vi "Setup PID.vi"() -> ()   [LabVIEW 2019]
uses:
  Controls/Global - Data UDP.vi
  Controls/UDP - Command.ctl
  Controls/Communication - Write Data.ctl
panel:
  in  "IP Address":string
  in  "Set":bool
  in  "Get":bool
  in  "Tab Control":enum32{"System", "Test", "ADC", "Sensor", "PID"}(tab)
  in  "System":string[][](table)=[["Out_Type"], ["Inverse"], ["Monitor"], ["ACC_Time"], ["Pulse_rev"], ["Stroke"], ["Auto Off"], ["Gear_Ratio"], ["Pitch"], ["Max Speed"], ["Jog Speed"], ["Disp Coff"], ["Max Load"]]
  in  "Test":string[][](table)=[["Traget #1"], ["Target #2"], ["Speed #1"], ["Speed #2"], [""], [""], [""], [""], [""], [""], [""], [""]]
  in  "ADC":string[][](table)=[["ActiveCH #0"], ["ActiveCH #1"], ["ActiveCH #2"], ["ActiveCH #3"], ["ActiveCH #4"], ["ActiveCH #5"], ["ActiveCH #6"], ["ActiveCH #7"], ["FilterType"], ["PostFilter #0"], ["PostFilter #1"], ["PostFilter #2"], ["PostFilter #3"], ["PostFilter #4"], ["PostFilter #5"], ["PostFilter #6"], ["PostFilter #7"], ["Gain #0"], ["Gain #1"], ["Gain #2"], ["Gain #3"], ["Gain #4"], ["Gain #5"], ["Gain #6"], ["Gain #7"], ["FS"], ["IntOC"], ["IntFC"], ["SysOC"], ["Cofficient #0"], ["Cofficient #1"], ["Cofficient #2"], ["Cofficient #3"], ["Cofficient #4"], ["Cofficient #5"], ["Cofficient #6"], ["Cofficient #7"], ["K1"], ["K2"], ["Max"]]
  in  "Sensor":string[][](table)=[["#1", ""], ["Name", ""], ["SUnit", ""], ["DecPoint", ""], ["Log", ""], ["H_Alarm", ""], ["L_Alarm", ""], ["H_Limit", ""], ["L_Limit", ""], ["Filter", ""], ["Gain", ""], ["Cal Type", " "], ["", ""], ["#2", ""], ["Name", ""], ["SUnit", ""], ["DecPoint", ""], ["Log", ""], ["H_Alarm", ""], ["L_Alarm", ""], ["H_Limit", ""], ["L_Limit", ""], ["Filter", ""], ["Gain", ""], ["Cal Type", ""], ["", ""], ["#3", ""], ["Name", ""], ["SUnit", ""], ["DecPoint", ""], ["Log", ""], ["H_Alarm", ""], ["L_Alarm", ""], ["H_Limit", ""], ["L_Limit", ""], ["Filter", ""], ["Gain", ""], ["Cal Type", ""], ["", ""], ["#4", ""], ["Name", ""], ["SUnit", ""], ["DecPoint", ""], ["Log", ""], ["H_Alarm", ""], ["L_Alarm", ""], ["H_Limit", ""], ["L_Limit", ""], ["Filter", ""], ["Gain", ""], ["Cal Type", ""]]
  in  "PID":string[][](table)=[["SP"], ["PV"], ["KP"], ["KI"], ["KD"], ["FF"], ["Err_Band"], ["Max"], ["Min"], ["Ts"], ["Out"], ["Mode"]]
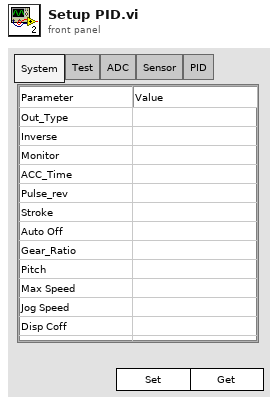
[diagram p1: front panel]
types:
  T1 = typedef "Communication - Write Data.ctl" = cluster{"Test":cluster{"Target Load":sgl, "Target Disp":sgl, "Rate":sgl, "Speed":sgl}, "Sensor":cluster{"Name":string[], "Unit":string[], "Decimal Point":u8[], "Ch Log":u8[], "H Alarm":u8[], "L Alarm":u8[], "H Limit":sgl[], "L Limit":sgl[], "Filter":u8[], "Gain":u8[], "Calib Type":u32[]}, "PID":cluster{"SP":sgl, "PV":sgl, "kP":sgl, "kI":sgl, "kD":sgl, "FF":sgl, "Err Band":sgl, "Max":i32, "Min":i32, "Ts":u32, "Out":i32, "Mode":u8}, "ADC":cluster{"Active Ch":u8[], "Filter Type":u8, "Post Filter":u8[], "Gain":u8[], "FS":u16, "IntOC":u8, "IntFC":u8, "SysOC":u8, "Cofficient":dbl[], "K":dbl[], "Max":i32}, "System":cluster{"Out Type":u8, "Inverse":u8, "Monitor":u8, "Reserve":u8, "ACC Time":u32, "Pulse Rev":u32, "Stroke":u32, "Auto Off":u32, "Gear Ratio":sgl, "Pitch":sgl, "Max Speed":u32, "Jog Speed":u32, "Disp Coff":sgl, "Max Load":u32}, "Index":enum16{"Ch1", "Ch2", "Ch3", "Ch4", "Ch5", "Ch6", "Ch7", "Ch8", "Ch9", "Ch10", "Ch11", "Ch12", "Ch13", "Ch14", "Ch15", "Ch16"}, "Datalog":enum16{"Ch1-Ch16", "Ch17-Ch32", "Ch32-Ch48", "Ch49-Ch64", "Empty"}}
  T2 = enum16{"Init", "Idle", "Get System", "Get Test", "Get ADC", "Get Sensor", "Get PID", "Set System", "Set Test", "Set ADC", "Set Sensor", "Set PID", "Exit"}
  T3 = typedef "UDP - Command.ctl" = enum16{"Stop", "Jog Up", "Jog Down", "Ramp Up", "Ramp Down", "PID Target", "PID Ramp", "Disp Run", "Read Ch Data", "Zero Channel", "Zero Disp", "Read Sensor", "Write Sensor", "Read ADC", "Write ADC", "Read PID", "Write PID", "Read Test", "Write Test", "Read System", "Write System", "Read Datalog", "Read Datalog Sensor"}
  T4 = cluster{"Out Type":u8, "Inverse":u8, "Monitor":u8, "Reserve":u8, "ACC Time":u32, "Pulse Rev":u32, "Stroke":u32, "Auto Off":u32, "Gear Ratio":sgl, "Pitch":sgl, "Max Speed":u32, "Jog Speed":u32, "Disp Coff":sgl, "Max Load":u32}
  T5 = cluster{"Out Type":string, "Inverse":string, "Monitor":string, "Reserve":string, "ACC Time":string, "Pulse Rev":string, "Stroke":string, "Auto Off":string, "Gear Ratio":string, "Pitch":string, "Max Speed":string, "Jog Speed":string, "Disp Coff":string, "Max Load":string}
  T6 = cluster{"Target Load":sgl, "Target Disp":sgl, "Rate":sgl, "Speed":sgl}
  T7 = cluster{"Target Load":string, "Target Disp":string, "Rate":string, "Speed":string}
  T8 = cluster{"Active Ch":u8[], "Filter Type":u8, "Post Filter":u8[], "Gain":u8[], "FS":u16, "IntOC":u8, "IntFC":u8, "SysOC":u8, "Cofficient":dbl[], "K":dbl[], "Max":i32}
  T9 = cluster{"Name":string[], "Unit":string[], "Decimal Point":u8[], "Ch Log":u8[], "H Alarm":u8[], "L Alarm":u8[], "H Limit":sgl[], "L Limit":sgl[], "Filter":u8[], "Gain":u8[], "Calib Type":u32[]}
  T10 = cluster{"SP":sgl, "PV":sgl, "kP":sgl, "kI":sgl, "kD":sgl, "FF":sgl, "Err Band":sgl, "Max":i32, "Min":i32, "Ts":u32, "Out":i32, "Mode":u8}
  T11 = cluster{"SP":string, "PV":string, "kP":string, "kI":string, "kD":string, "FF":string, "Err Band":string, "Max":string, "Min":string, "Ts":string, "Out":string, "Mode":string}
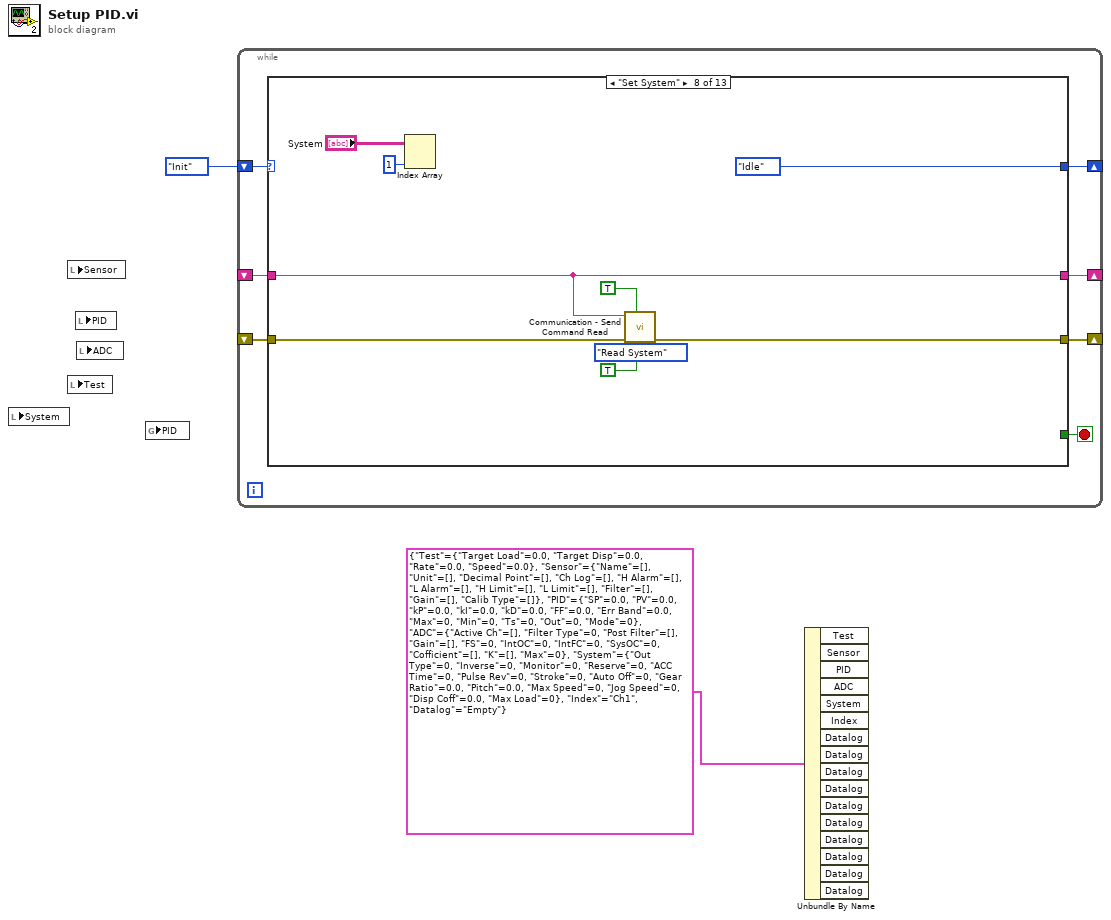
[diagram p0: block diagram]
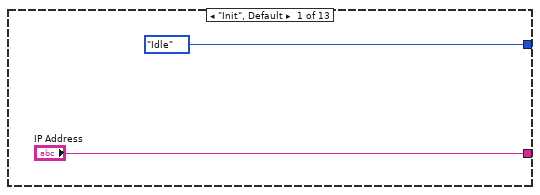
[diagram p2: hidden frame]
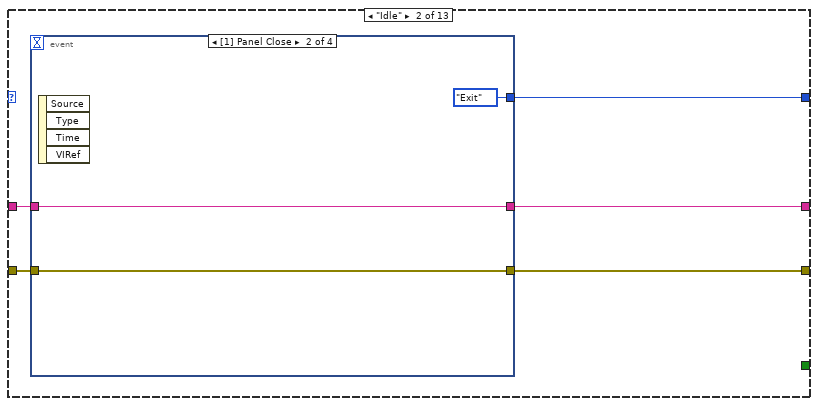
[diagram p3: hidden frame]
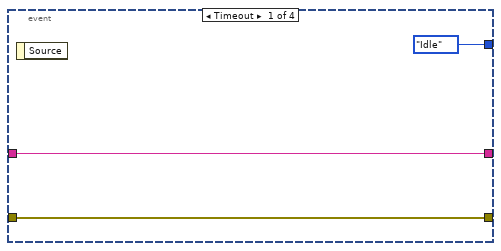
[diagram p4: hidden frame]
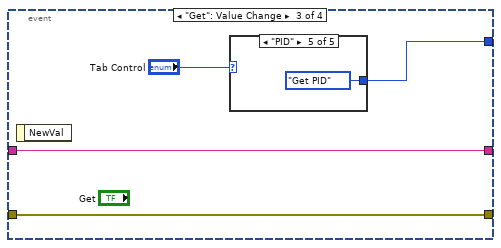
[diagram p5: hidden frame]
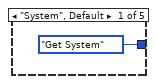
[diagram p6: hidden frame]
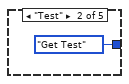
[diagram p7: hidden frame]
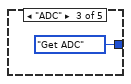
[diagram p8: hidden frame]
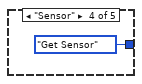
[diagram p9: hidden frame]
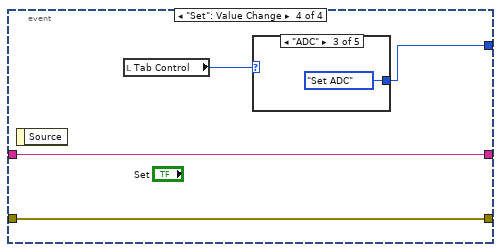
[diagram p10: hidden frame]
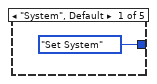
[diagram p11: hidden frame]
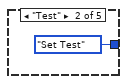
[diagram p12: hidden frame]
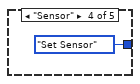
[diagram p13: hidden frame]
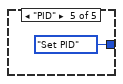
[diagram p14: hidden frame]
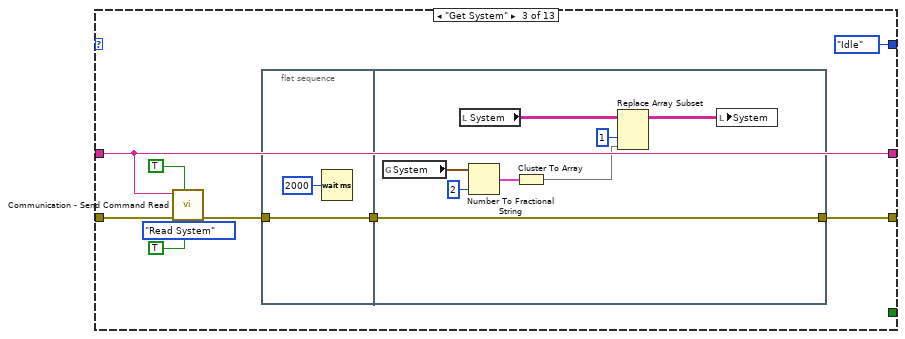
[diagram p15: hidden frame]
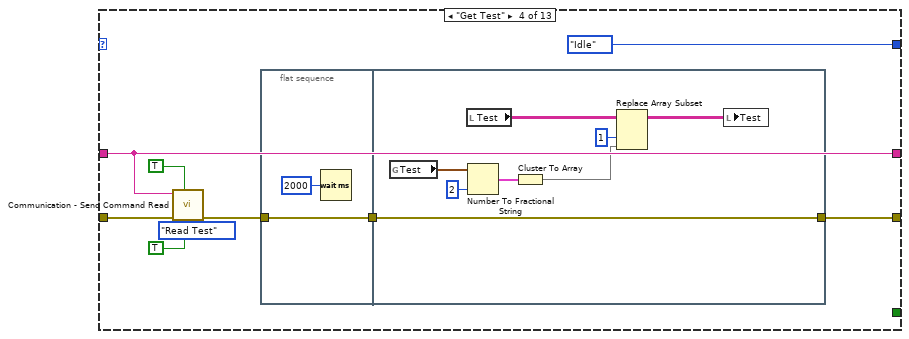
[diagram p16: hidden frame]
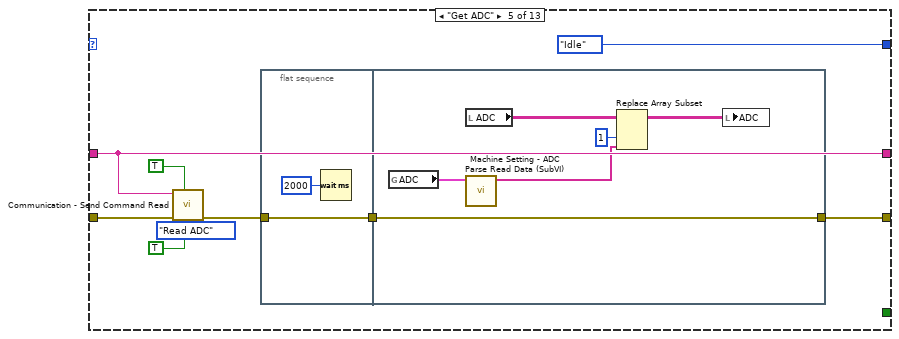
[diagram p17: hidden frame]
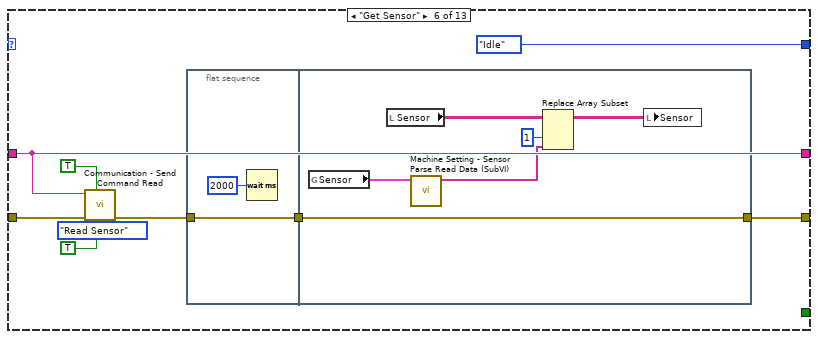
[diagram p18: hidden frame]
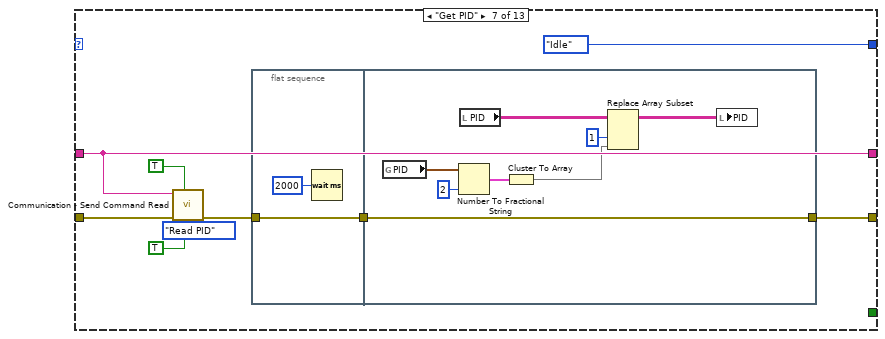
[diagram p19: hidden frame]
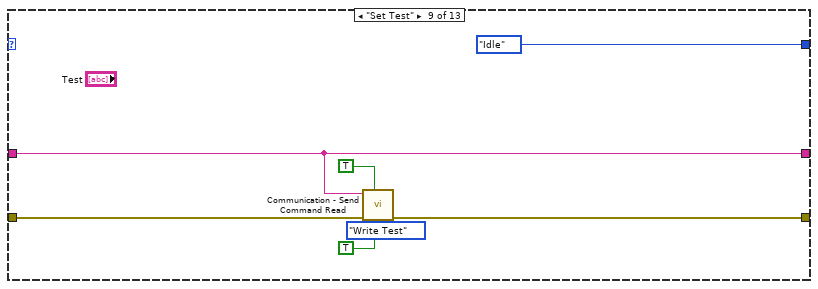
[diagram p20: hidden frame]
diagram:
  n1 = local read "System"() -> ()  [unwired: 1 in]
  n2 = local read "Sensor"() -> ()  [unwired: 1 in]
  n3 = local read "Test"() -> ()  [unwired: 1 in]
  n4 = local read "PID"() -> ()  [unwired: 1 in]
  n5 = local read "ADC"() -> ()  [unwired: 1 in]
  n6 = global read "Global - Data UDP.vi" "PID"() -> ()  [unwired: 1 in]
  n7 = while {
    shift-right: [w8] -> _
    shift-left: T2."Init" -> [w9]
    shift-right: [w6] -> _
    shift-left: _ -> [w5]
    shift-right: [w4] -> _
    shift-left: _ -> [w3]
    stop <- w7 stop-if-true
    n8 = case shown="\"Set System\"" w9 {
      tunnel: [T2."Idle" w16 T2."Idle" T2."Idle" T2."Idle" T2."Idle" T2."Idle" T2."Idle" T2."Idle" T2."Idle" T2."Idle" T2."Idle" T2."Exit"] -> w8
      tunnel: [_ _ _ _ _ _ _ _ _ _ _ _ TRUE] -> w7
      tunnel: ["IP Address" w14 w46 w63 w82 w99 w116 w134 w141 w148 w155 w162 "" ("IP Address")] -> w6
      tunnel: w5 -> [_ w15 w46 w63 w82 w99 w116 w134 w141 w148 w155 w162 _]
      tunnel: [_ w13 w43 w60 w79 w96 w113 w135 w142 w149 w156 w163 _] -> w4
      tunnel: w3 -> [_ w12 w47 w64 w83 w100 w117 w136 w143 w150 w157 w164 _]
      frame "Init", Default {
      }
      frame "Idle" {
        n9 = event shown="[1] Panel Close" {
          selector: _ -> [_ _ _ _]
          dyn-events: _ -> [_ _ _ _]
          timeout: _ -> [_ _ _ _]
          tunnel: [T2."Idle" T2."Exit" w25 w34] -> w16
          tunnel: w15 -> [w18 w22 w24 w33]
          tunnel: [w18 w22 w24 w33] -> w14
          tunnel: [w17 w20 w23 w32] -> w13
          tunnel: w12 -> [w17 w20 w23 w32]
          event Timeout {
            n10 = event-data() -> ()  [unwired: 1 in, 1 out]
          }
          event Panel Close {
            n11 = event-data() -> ()  [unwired: 1 in, 4 out]
          }
          event "Get": Value Change {
            n12 = event-data() -> ()  [unwired: 1 in, 1 out]
            n13 = case shown="\"PID\"" "Tab Control" {
              tunnel: [T2."Get System" T2."Get Test" T2."Get ADC" T2."Get Sensor" T2."Get PID"] -> w25
              frame "System", Default {
              }
              frame "Test" {
              }
              frame "ADC" {
              }
              frame "Sensor" {
              }
              frame "PID" {
              }
            }
          }
          event "Set": Value Change {
            n14 = event-data() -> ()  [unwired: 1 in, 1 out]
            n15 = local read "Tab Control"() -> (w35:enum32{"System", "Test", "ADC", "Sensor", "PID"})
            n16 = case shown="\"ADC\"" w35 {
              tunnel: [T2."Set System" T2."Set Test" T2."Set ADC" T2."Set Sensor" T2."Set PID"] -> w34
              frame "System", Default {
              }
              frame "Test" {
              }
              frame "ADC" {
              }
              frame "Sensor" {
              }
              frame "PID" {
              }
            }
          }
        }
      }
      frame "Get System" {
        n17 = call "Communication - Send Command Read.vi"("Fron?"=TRUE, "Bypass?"=TRUE, "error in (no error)"=w47, "Action"=UDP_-_Command."Read System", "Device IP Address"=w46) -> ("error out"=w41:errorcluster)  [unwired: 6 in]
        n18 = flat-sequence {
          tunnel: [w50] -> w42
          tunnel: w41 -> [w50]
          tunnel: [w52] -> w43
          tunnel: w42 -> [w52]
          frame #0 {
            n19 = Wait (ms)(milliseconds to wait=u32 2000) -> ()  [unwired: 1 out]
          }
          frame #1 {
            n20 = global read "Global - Data UDP.vi" "System"() -> (w56:T4)
            n21 = local read "System"() -> (w59:string[][])
            n22 = Number To Fractional String(number=w56, precision (6)=i16 2) -> (F-format string=w54:T5)  [unwired: 2 in]
            n23 = Cluster To Array(cluster=w54) -> (array=w53:string[])
            n24 = Replace Array Subset(array=w59, new element=w53, index (col)=1 ("disabled index (col)")) -> (w58:string[][])  [unwired: 1 in]
            n25 = local write "System"(w58) -> ()
          }
        }
      }
      frame "Get Test" {
        n26 = call "Communication - Send Command Read.vi"("Fron?"=TRUE, "Bypass?"=TRUE, "error in (no error)"=w64, "Action"=UDP_-_Command."Read Test", "Device IP Address"=w63) -> ("error out"=w61:errorcluster)  [unwired: 6 in]
        n27 = flat-sequence {
          tunnel: [w69] -> w62
          tunnel: w61 -> [w69]
          tunnel: [w71] -> w60
          tunnel: w62 -> [w71]
          frame #0 {
            n28 = Wait (ms)(milliseconds to wait=u32 2000) -> ()  [unwired: 1 out]
          }
          frame #1 {
            n29 = global read "Global - Data UDP.vi" "Test"() -> (w75:T6)
            n30 = local read "Test"() -> (w78:string[][])
            n31 = Number To Fractional String(number=w75, precision (6)=i16 2) -> (F-format string=w73:T7)  [unwired: 2 in]
            n32 = Cluster To Array(cluster=w73) -> (array=w72:string[])
            n33 = Replace Array Subset(array=w78, new element=w72, index (col)=1 ("disabled index (col)")) -> (w77:string[][])  [unwired: 1 in]
            n34 = local write "Test"(w77) -> ()
          }
        }
      }
      frame "Get ADC" {
        n35 = call "Communication - Send Command Read.vi"("Fron?"=TRUE, "Bypass?"=TRUE, "error in (no error)"=w83, "Action"=UDP_-_Command."Read ADC", "Device IP Address"=w82) -> ("error out"=w80:errorcluster)  [unwired: 6 in]
        n36 = flat-sequence {
          tunnel: [w88] -> w81
          tunnel: w80 -> [w88]
          tunnel: [w92] -> w79
          tunnel: w81 -> [w92]
          frame #0 {
            n37 = Wait (ms)(milliseconds to wait=u32 2000) -> ()  [unwired: 1 out]
          }
          frame #1 {
            n38 = global read "Global - Data UDP.vi" "ADC"() -> (w91:T8)
            n39 = local read "ADC"() -> (w95:string[][])
            n40 = call "Machine Setting - ADC Parse Read Data (SubVI).vi"("ADC"=w91) -> ("Array"=w90:string[])  [unwired: 10 in]
            n41 = Replace Array Subset(array=w95, new element=w90, index (col)=1 ("disabled index (col)")) -> (w94:string[][])  [unwired: 1 in]
            n42 = local write "ADC"(w94) -> ()
          }
        }
      }
      frame "Get Sensor" {
        n43 = call "Communication - Send Command Read.vi"("Fron?"=TRUE, "Bypass?"=TRUE, "error in (no error)"=w100, "Action"=UDP_-_Command."Read Sensor", "Device IP Address"=w99) -> ("error out"=w97:errorcluster)  [unwired: 6 in]
        n44 = flat-sequence {
          tunnel: [w105] -> w98
          tunnel: w97 -> [w105]
          tunnel: [w109] -> w96
          tunnel: w98 -> [w109]
          frame #0 {
            n45 = Wait (ms)(milliseconds to wait=u32 2000) -> ()  [unwired: 1 out]
          }
          frame #1 {
            n46 = global read "Global - Data UDP.vi" "Sensor"() -> (w108:T9)
            n47 = local read "Sensor"() -> (w112:string[][])
            n48 = call "Machine Setting - Sensor Parse Read Data (SubVI).vi"("Sensor"=w108) -> ("Array"=w107:string[])  [unwired: 10 in]
            n49 = Replace Array Subset(array=w112, new element=w107, index (col)=1 ("disabled index (col)")) -> (w111:string[][])  [unwired: 1 in]
            n50 = local write "Sensor"(w111) -> ()
          }
        }
      }
      frame "Get PID" {
        n51 = call "Communication - Send Command Read.vi"("Fron?"=TRUE, "Bypass?"=TRUE, "error in (no error)"=w117, "Action"=UDP_-_Command."Read PID", "Device IP Address"=w116) -> ("error out"=w114:errorcluster)  [unwired: 6 in]
        n52 = flat-sequence {
          tunnel: [w122] -> w115
          tunnel: w114 -> [w122]
          tunnel: [w124] -> w113
          tunnel: w115 -> [w124]
          frame #0 {
            n53 = Wait (ms)(milliseconds to wait=u32 2000) -> ()  [unwired: 1 out]
          }
          frame #1 {
            n54 = global read "Global - Data UDP.vi" "PID"() -> (w128:T10)
            n55 = Number To Fractional String(number=w128, precision (6)=i16 2) -> (F-format string=w126:T11)  [unwired: 2 in]
            n56 = local read "PID"() -> (w131:string[][])
            n57 = Cluster To Array(cluster=w126) -> (array=w125:string[])
            n58 = Replace Array Subset(array=w131, new element=w125, index (col)=1 ("disabled index (col)")) -> (w130:string[][])  [unwired: 1 in]
            n59 = local write "PID"(w130) -> ()
          }
        }
      }
      frame "Set System" {
        n60 = Index Array(array="System", index (col)=1 ("disabled index (col)")) -> ()  [unwired: 1 in, 1 out]
        n61 = call "Communication - Send Command Read.vi"("Fron?"=TRUE, "Bypass?"=TRUE, "error in (no error)"=w136, "Action"=UDP_-_Command."Read System", "Device IP Address"=w134) -> ("error out"=w135:errorcluster)  [unwired: 6 in]
      }
      frame "Set Test" {
        n62 = call "Communication - Send Command Read.vi"("Fron?"=TRUE, "Bypass?"=TRUE, "error in (no error)"=w143, "Action"=UDP_-_Command."Write Test", "Device IP Address"=w141) -> ("error out"=w142:errorcluster)  [unwired: 6 in]
      }
      frame "Set ADC" {
        n63 = call "Communication - Send Command Read.vi"("Fron?"=TRUE, "Bypass?"=TRUE, "error in (no error)"=w150, "Action"=UDP_-_Command."Write ADC", "Device IP Address"=w148) -> ("error out"=w149:errorcluster)  [unwired: 6 in]
      }
      frame "Set Sensor" {
        n64 = call "Communication - Send Command Read.vi"("Fron?"=TRUE, "Bypass?"=TRUE, "error in (no error)"=w157, "Action"=UDP_-_Command."Write Sensor", "Device IP Address"=w155) -> ("error out"=w156:errorcluster)  [unwired: 6 in]
      }
      frame "Set PID" {
        n65 = call "Communication - Send Command Read.vi"("Fron?"=TRUE, "Bypass?"=TRUE, "error in (no error)"=w164, "Action"=UDP_-_Command."Write PID", "Device IP Address"=w162) -> ("error out"=w163:errorcluster)  [unwired: 6 in]
      }
      frame "Exit" {
      }
    }
  }
  n66 = Unbundle By Name(T1 {"Test"={"Target Load"=0.0, "Target Disp"=0.0, "Rate"=0.0, "Speed"=0.0}, "Sensor"={"Name"=[], "Unit"=[], "Decimal Point"=[], "Ch Log"=[], "H Alarm"=[], "L Alarm"=[], "H Limit"=[], "L Limit"=[], "Filter"=[], "Gain"=[], "Calib Type"=[]}, "PID"={"SP"=0.0, "PV"=0.0, "kP"=0.0, "kI"=0.0, "kD"=0.0, "FF"=0.0, "Err Band"=0.0, "Max"=0, "Min"=0, "Ts"=0, "Out"=0, "Mode"=0}, "ADC"={"Active Ch"=[], "Filter Type"=0, "Post Filter"=[], "Gain"=[], "FS"=0, "IntOC"=0, "IntFC"=0, "SysOC"=0, "Cofficient"=[], "K"=[], "Max"=0}, "System"={"Out Type"=0, "Inverse"=0, "Monitor"=0, "Reserve"=0, "ACC Time"=0, "Pulse Rev"=0, "Stroke"=0, "Auto Off"=0, "Gear Ratio"=0.0, "Pitch"=0.0, "Max Speed"=0, "Jog Speed"=0, "Disp Coff"=0.0, "Max Load"=0}, "Index"=enum."Ch1", "Datalog"=enum."Empty"} ("Data")) -> ()  [unwired: 16 out]
